vi "Initialize.vi"(7 "Serial Configuration":T1={"Baud Rate"=9600, "Parity"=0, "Data Bits"=8, "Stop Bits"=10, "Flow Control"=0} {"Flow Control" items=["None", "XON/XOFF", "RTS/CTS", "XON/XOFF & RTS/CTS", "DTR/DSR", "XON/XOFF & DTR/DSR"]; "Stop Bits" items=["1.0"=10, "1.5"=15, "2.0"=20]; "Data Bits" items=["7"=7, "8"=8]; "Parity" items=["None", "Odd", "Even", "Mark", "Space"]; "Baud Rate" items=["300"=300, "600"=600, "1200"=1200, "2400"=2400, "4800"=4800, "9600"=9600, "19200"=19200]}, 8 "error in (no error)":errorcluster, 9 "Reset (True)":bool=TRUE, 10 "ID Query (True)":bool=TRUE, 11 "VISA resource name":refnum<visa-resource-name>) -> (0 "error out":errorcluster, 3 "VISA resource name out":refnum<visa-resource-name>)   [LabVIEW 2012, in "Temptronic TP04300.lvlib"]
doc: "Establishes communication with the instrument and optionally performs an instrument identification query and/or an instrument reset. It also places the instrument in a default state needed for other instrument driver operations. Therefore, call this VI before calling other instrument driver VIs for this instrument. Generally, you need to call the <B>Initialize VI</B> only once at the beginning of an application."
uses:
  <instrlib>/Temptronic TP04300/Temptronic TP04300.lvlib
panel:
  # "© 2007 Temptronic Corporation.  ALL RIGHTS RESERVED."
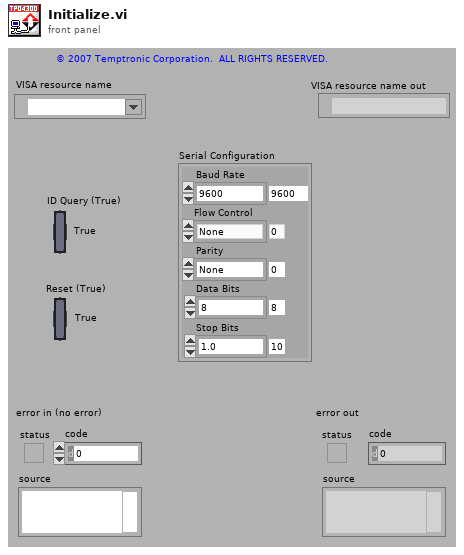
[diagram p1: front panel]
types:
  T1 = cluster{"Baud Rate":u32, "Parity":u16, "Data Bits":u16, "Stop Bits":u16, "Flow Control":u16}
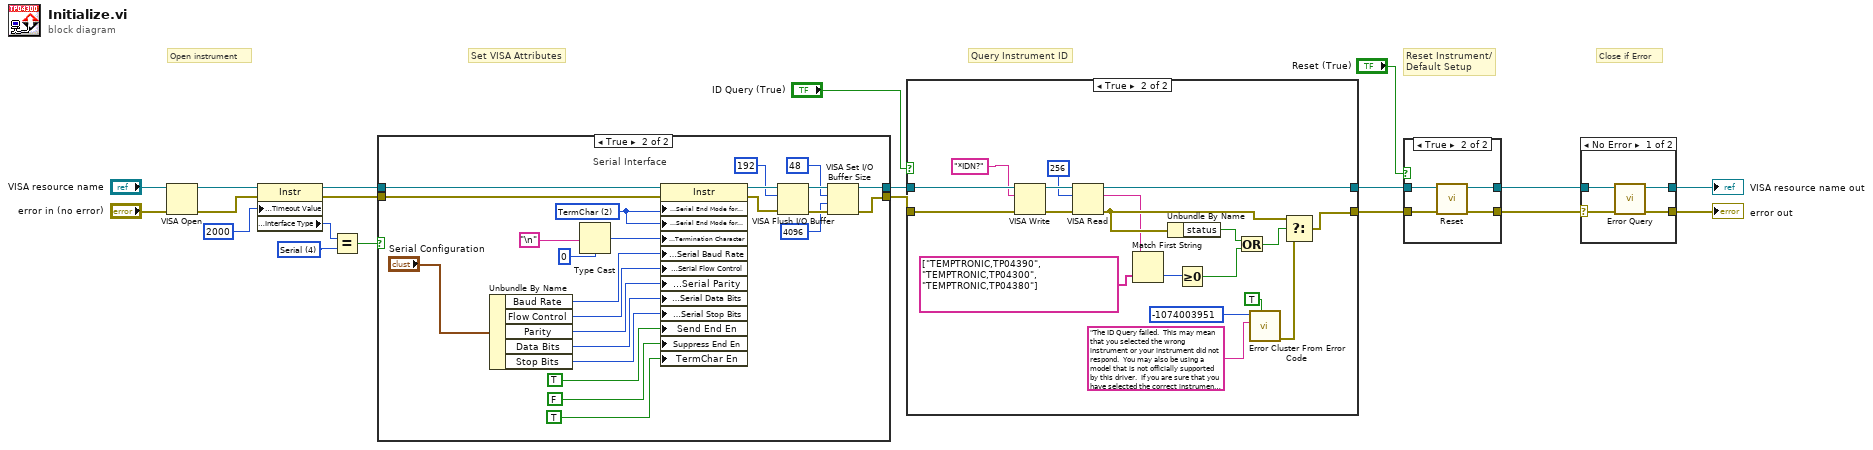
[diagram p0: block diagram]
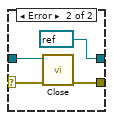
[diagram p3: hidden frame]
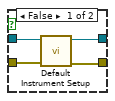
[diagram p4: hidden frame]
diagram:
  w8 = u16 4 items=["GPIB"=1, "VXI"=2, "GPIB-VXI"=3, "Serial"=4, "PXI"=5, "TCPIP"=6, "USB"=7] ("Interface Information:Interface Type")
  # "Set VISA Attributes"
  # "Close if Error"
  # "Query Instrument ID"
  # "Reset Instrument/\nDefault Setup"
  # "Open instrument"
  n1 = VISA Open(error in (no error)="error in (no error)", VISA resource name="VISA resource name") -> (VISA resource name=w2:refnum<visa-resource-name>, error out=w3:errorcluster)  [unwired: 3 in]
  n2 = property class="Instr"(reference=w2, error in=w3, "General Settings:Timeout Value"=u32 2000) -> (reference out=w10:refnum<visa-resource-name>, error out=w9:errorcluster, "Interface Information:Interface Type"=w14:u16)
  n3 = Equal?(x=w14, y=w8) -> (x = y?=w1:bool)
  n4 = case shown="True" w1 {
    tunnel: [w21 w43] -> w12
    tunnel: [w22 w40] -> w11
    tunnel: w10 -> [w21 w45]
    tunnel: w9 -> [w22 w46]
    frame False {
      # "GPIB and TCP/IP Interface"
    }
    frame True {
      w23 = u16 2 items=["None", "Last Bit", "TermChar", "Break"] ("Serial Settings:End Mode for Writes")
      # "Serial Interface"
      n5 = Unbundle By Name("Serial Configuration") -> ("Baud Rate"=w33:u32, "Flow Control"=w29:u16, "Parity"=w31:u16, "Data Bits"=w32:u16, "Stop Bits"=w28:u16)
      n6 = Type Cast(type=u8 0, x="\n") -> (*(type *) &x=w34:u8)
      n7 = property class="Instr"(reference=w45, error in=w46, "Serial Settings:Serial End Mode for Reads"=w23, "Serial Settings:Serial End Mode for Writes"=w23, "Message Based Settings:Termination Character"=w34, "Serial Settings:Serial Baud Rate"=w33, "Serial Settings:Serial Flow Control"=w29, "Serial Settings:Serial Parity"=w31, "Serial Settings:Serial Data Bits"=w32, "Serial Settings:Serial Stop Bits"=w28, "Send End En"=TRUE, "Suppress End En"=FALSE, "TermChar En"=TRUE) -> (reference out=w39:refnum<visa-resource-name>, error out=w42:errorcluster)
      n8 = VISA Flush I/O Buffer(VISA resource name=w39, mask (16)=u16 192, error in (no error)=w42) -> (VISA resource name out=w44:refnum<visa-resource-name>, error out=w41:errorcluster)
      n9 = VISA Set I/O Buffer Size(VISA resource name=w44, mask (16)=u16 48, size (4096)=u32 4096 ("size (0)"), error in (no error)=w41) -> (VISA resource name out=w43:refnum<visa-resource-name>, error out=w40:errorcluster)
    }
  }
  n10 = case shown="True" "ID Query (True)" {
    tunnel: [w47 w52] -> w19
    tunnel: [w48 w65] -> w20
    tunnel: w12 -> [w48 w66]
    tunnel: w11 -> [w47 w67]
    frame False {
    }
    frame True {
      n11 = VISA Write(VISA resource name=w66, write buffer="*IDN?", error in (no error)=w67) -> (VISA resource name out=w64:refnum<visa-resource-name>, error out=w63:errorcluster)  [unwired: 1 out]
      n12 = VISA Read(VISA resource name=w64, byte count=u32 256, error in (no error)=w63) -> (VISA resource name out=w65:refnum<visa-resource-name>, read buffer=w51:string, error out=w54:errorcluster)  [unwired: 1 out]
      n13 = Match First String(2:string[] ["TEMPTRONIC,TP04390", "TEMPTRONIC,TP04300", "TEMPTRONIC,TP04380"] ("string array"), 3:w51) -> (0:w49:i32)  [unwired: 1 out]
      n14 = Unbundle By Name(w54) -> ("status"=w59:bool)
      n15 = Greater Or Equal To 0?(x=w49) -> (x >= 0?=w60:bool)
      n16 = Or(x=w59, y=w60) -> (x .or. y?=w53:bool)
      n17 = call <vilib>:"Error Cluster From Error Code.vi"("show call chain? (False)"=TRUE, "error message (\"\")"="The ID Query failed.  This may mean that you selected the wrong instrument or your instrument did not respond.  You may also be using a model that is not officially supported by this driver.  If you are sure that you have selected the correct instrument and it is responding, try disabling the ID Query." ("Source (VI Name)"), "error code (0)"=-1074003951 ("Code")) -> ("error out"=w55:errorcluster)  [unwired: 6 in]
      n18 = Select(t=w54, s=w53, f=w55) -> (s? t:f=w52:errorcluster)
    }
  }
  n19 = case shown="True" "Reset (True)" {
    tunnel: w19 -> [w71 w72]
    tunnel: [w70 w75] -> w4
    tunnel: w20 -> [w68 w73]
    tunnel: [w69 w74] -> w5
    frame False {
      n20 = call <instrlib>:"Default Instrument Setup.vi"("error in (no error)"=w71, "VISA resource name"=w68) -> ("error out"=w70:errorcluster, "VISA resource name out"=w69:refnum<visa-resource-name>)  [unwired: 8 in]
    }
    frame True {
      n21 = call <instrlib>:"Reset.vi"("error in (no error)"=w72, "VISA resource name"=w73) -> ("error out"=w75:errorcluster, "VISA resource name out"=w74:refnum<visa-resource-name>)  [unwired: 8 in]
    }
  }
  n22 = case shown="No Error" w4 {
    selector: w4 -> [w77 w81]
    tunnel: w5 -> [w76 w82]
    tunnel: [w79 refnum<visa-resource-name> refnum ("VISA resource name out")] -> w7
    tunnel: [w78 w83] -> w6
    frame No Error {
      n23 = call <instrlib>:"Error Query.vi"("error in (no error)"=w77, "VISA resource name"=w76) -> ("error out"=w78:errorcluster, "VISA resource name out"=w79:refnum<visa-resource-name>)  [unwired: 6 in, 2 out]
    }
    frame Error {
      n24 = call <instrlib>:"Close.vi"("error in (no error)"=w81, "VISA resource name"=w82) -> ("error out"=w83:errorcluster)  [unwired: 9 in]
    }
  }
  "VISA resource name out" <- w7
  "error out" <- w6
